vi "Stage Enforce Limits.vi"(6 "Lane separation (mm)":dbl min=0.0 step=0.001, 7 "Forward step (mm)":dbl min=0.0 step=0.001, 8 "error in (no error)":errorcluster, 10 "Enforce software stage limits":bool=TRUE, 11 "Application in":refnum<class "Application.lvclass">) -> (0 "error out":errorcluster, 3 "Application out":refnum<class "Application.lvclass">)   [LabVIEW 2023, in "Application.lvlib" / "Application.lvclass"]
uses:
  Application.lvclass
  Application.lvclass/Application.ctl
  Hardware/Stage Controller Messages/Enforce Limits Msg/Enforce Limits Msg.lvclass
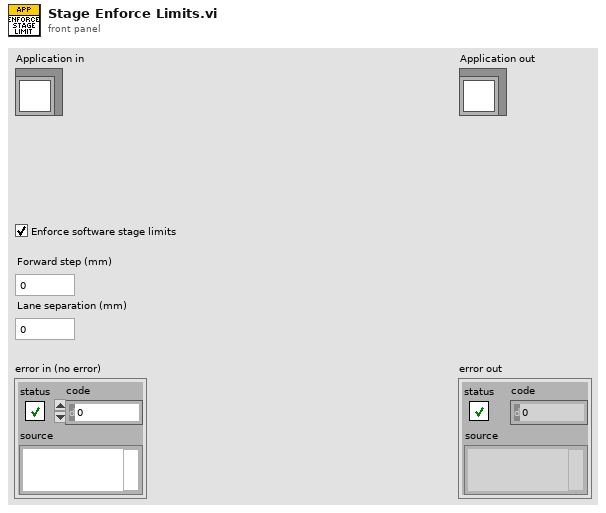
[diagram p1: front panel]
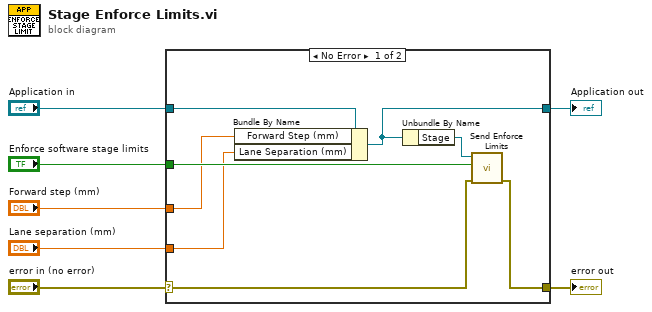
[diagram p0: block diagram]
diagram:
  n1 = case shown="No Error" "error in (no error)" {
    selector: "error in (no error)" -> [w14 w17]
    tunnel: [w13 w17] -> w6
    tunnel: [w10 w16] -> w4
    tunnel: "Application in" -> [w11 w16]
    tunnel: "Enforce software stage limits" -> [w12 _]
    tunnel: "Forward step (mm)" -> [w8 _]
    tunnel: "Lane separation (mm)" -> [w9 _]
    frame No Error {
      n2 = Bundle By Name(cluster=w11, "Forward Step (mm)"=w8, "Lane Separation (mm)"=w9) -> (w10:refnum<class "Application.lvclass">)
      n3 = Unbundle By Name(w10) -> ("Stage"=w15:refnum<class "Message Enqueuer.lvclass">)
      n4 = call "Send Enforce Limits.vi"("error in (no error)"=w14, "Enforce software stage limits"=w12, "Message Enqueuer"=w15) -> ("error out"=w13:errorcluster)  [unwired: 7 in, 1 out]
    }
    frame Error {
    }
  }
  "error out" <- w6
  "Application out" <- w4
